vi "LJM_eReadNames.vi"(0 "Handle In":i32, 1 "NumFrames (Auto-Detect)":i32=-1, 5 "aNames":string[](array[string]), 11 "error in":errorcluster) -> (4 "Handle Out":i32, 10 "aValuesOut":dbl[](array[numeric]) format="%.2f", 14 "ErrorAddress":i32, 15 "error out":errorcluster)   [LabVIEW 2026]
panel:
  # "1/20/2015:  Default value of NumFrames changed to -1 which\nequates to Auto-Detect.  If NumFrames = -1, then the NumFrames\ncontrol is ignored and the size of aNames/aAddresses is used to\ndetermine how many frames there are."
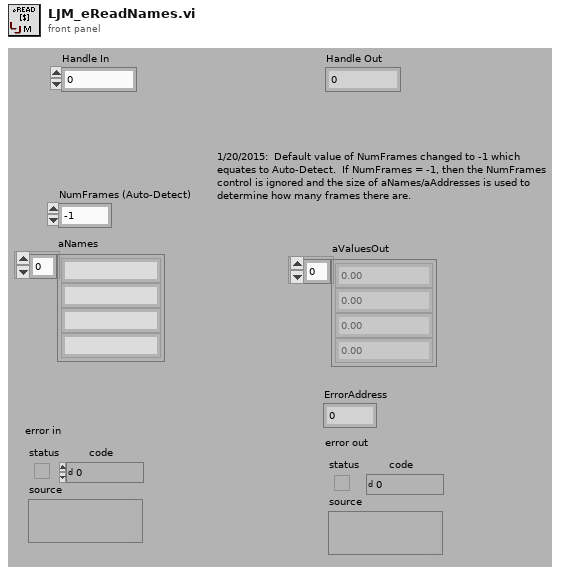
[diagram p1: front panel]
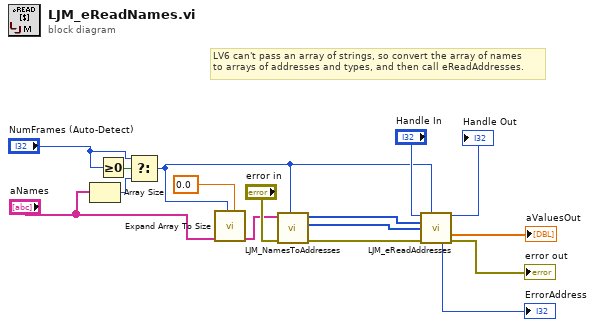
[diagram p0: block diagram]
diagram:
  # "LV6 can't pass an array of strings, so convert the array of names\nto arrays of addresses and types, and then call eReadAddresses."
  n1 = Array Size(array="aNames") -> (size(s)=w5:i32)
  n2 = Greater Or Equal To 0?(x="NumFrames (Auto-Detect)") -> (x >= 0?=w4:bool)
  n3 = Select(t="NumFrames (Auto-Detect)", s=w4, f=w5) -> (s? t:f=w1:i32)
  n4 = call "Expand Array To Size.vi"("Default Value"=0.0, "# Elements"=w1, "String Array In"="aNames") -> ("String Array Out"=w15:string[])  [unwired: 4 in, 4 out]
  n5 = call "LJM_NamesToAddresses.vi"("NumFrames (Auto-Detect)"=w1, "error in"="error in", "aNames"=w15) -> ("error out"=w13:errorcluster, "aTypes"=w11:i32[], "aAddresses"=w12:i32[])  [unwired: 6 in]
  n6 = call "LJM_eReadAddresses.vi"("Handle In"="Handle In", "NumFrames (Auto-Detect)"=w1, "aAddresses"=w12, "aTypes"=w11, "error in"=w13) -> ("Handle Out"=→"Handle Out":i32, "aValues"=→"aValuesOut":dbl[], "ErrorAddress"=→"ErrorAddress":i32, "error out"=→"error out":errorcluster)  [unwired: 7 in]
